vi "Wait on chirps generation - sweep.vi"(8 "error in (no error)":errorcluster) -> (0 "error out":errorcluster, 3 "Timed out waiting on Chirps generation":bool)   [LabVIEW 2017]
uses:
  Typedefs/Set Main VI cursor.ctl
  Global Variables/gl_UI Ctrl Refs.vi
  Global Variables/General Globals.vi
panel:
  out "Elapsed Time (s)":dbl
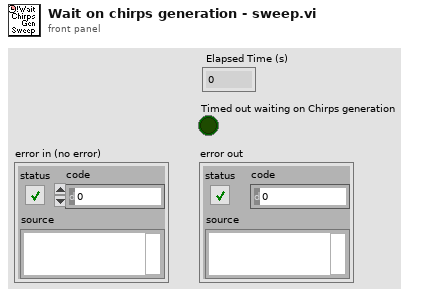
[diagram p1: front panel]
types:
  T1 = typedef "Set Main VI cursor.ctl" = enum16{"Release busy cursor", "Set busy cursor"}
  T2 = typedef "UI ctrl refs cluster.ctl" = cluster{"Top level VI path":path, "Top level VI ref":refnum<vi>, "User menu ref":refnum<k9>, "Sub Panel control":refnum<vi>, "Imaging Param Tab":refnum<vi>, "Occurrence-Start drivers":refnum<k4>, "Occurrence-Speed logging initialised":refnum<k4>, "Occurrence-XYZ stage initialised":refnum<k4>, "Exit button":refnum<vi>, "Status ind":refnum<vi>, "Set as origin":refnum<vi>, "Speed Logging":refnum<vi>, "Time Lapse":refnum<vi>, "Live Imaging":refnum<vi>, "AOL Z Stack":refnum<vi>, "Motor Z Stack":refnum<vi>, "Funct Acq button":refnum<vi>, "Hard Shutter":refnum<vi>, "Virtual Shutter":refnum<vi>, "Laser Power":refnum<vi>, "AOL Mode":refnum<vi>, "Frame Size":refnum<vi>, "Field of View":refnum<vi>, "Dwell Time":refnum<vi>, "Zoom":refnum<vi>, "AOL Z":refnum<vi>, "Objective":refnum<vi>, "Axis":refnum<vi>, "Paths & Names":refnum<vi>, "Experiment folder path (ind.)":refnum<vi>, "Last State (Ind.)":refnum<vi>, "Averages":refnum<vi>, "Angle (degrees)":refnum<vi>, "X centre":refnum<vi>, "Y centre":refnum<vi>, "Plane Mode":refnum<vi>, "# Planes":refnum<vi>, "Z Start":refnum<vi>, "Z Stop":refnum<vi>, "Z Step":refnum<vi>, "PMT 1":refnum<vi>, "PMT 2":refnum<vi>, "Stage XYZ Position":refnum<vi>, "Pockels@Z Start":refnum<vi>, "Pockels@Z Stop":refnum<vi>, "Obtain Z Start":refnum<vi>, "Obtain Z Stop":refnum<vi>, "Live stim.trig.period":refnum<vi>, "Live stim.trig.enable":refnum<vi>, "Movement Correction":refnum<vi>, "Load Reference Image":refnum<vi>, "XY Stage Move":refnum<vi>, "MovCor Cluster":refnum<vi>, "RefDAQParam":refnum<vi>, "Funct. Acq. Pockels Modulation":refnum<vi>, "Ref Laser Power":refnum<vi>, "Enable Video Recording":refnum<vi>, "Video Record-Live Imaging":refnum<vi>, "Video Record-Funct acq":refnum<vi>, "Reference Source":refnum<vi>, "AOL Z-stack Chirps Ready (ind)":refnum<vi>, "Target time between mov.cor. ref triggers (ms)":refnum<vi>, "Funct. Acq. Ref frame save":refnum<vi>, "Tracking button":refnum<vi>, "Show ref plots window":refnum<vi>, "Center freq ind (nm)":refnum<vi>, "Pickup mode (ind)":refnum<vi>, "Logging queue (ind)":refnum<vi>, "Back aperture power (ind.)":refnum<vi>, "Power after objective (ind.)":refnum<vi>, "Switch user":refnum<vi>, "Ls1 Conn. Status":refnum<vi>, "Ls1Tuning Status":refnum<vi>, "Ls1 Faults":refnum<vi>, "Ls1 Connection":refnum<vi>, "Ls1 Mode":refnum<vi>, "Ls1 POWER [mW]":refnum<vi>, "Ls1Shutter":refnum<vi>, "Ls1 Wavelength":refnum<vi>, "Ls1 Note":refnum<vi>, "Ls1 Confirm Wav":refnum<vi>, "Ls1 PreChrp Prism1":refnum<vi>, "Ls1 PreChrp Prism2":refnum<vi>, "Ls1 wav top Ind":refnum<vi>, "Ls1 power top Ind":refnum<vi>, "Ls1 Pump peak Hold":refnum<vi>, "Ls1 Status Ind":refnum<vi>, "Ls1 wav cancel":refnum<vi>, "Experiment Type":refnum<vi>, "Biology Information":refnum<vi>, "Camera recording status":refnum<vi>, "Start Sweep":refnum<vi>, "# Sw. Planes":refnum<vi>}
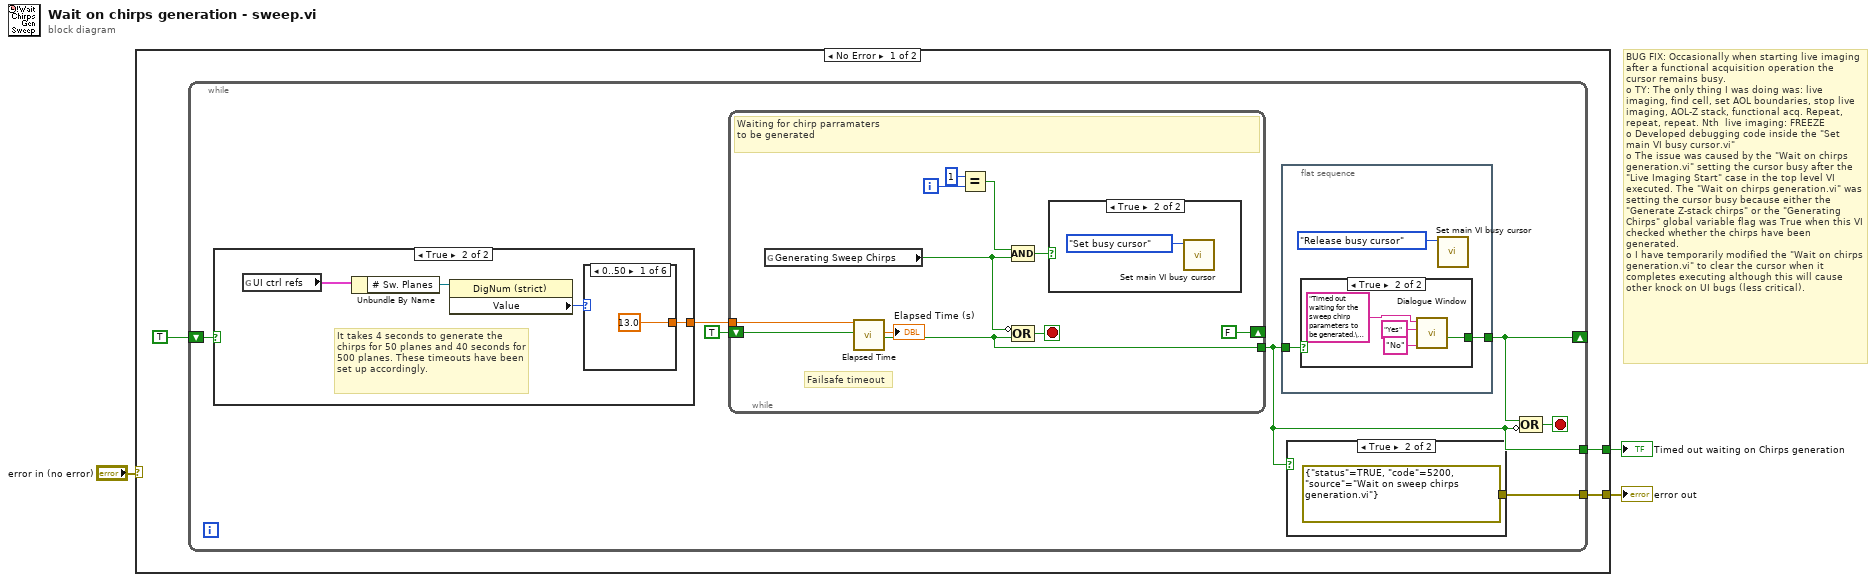
[diagram p0: block diagram]
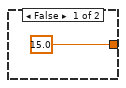
[diagram p3: hidden frame]
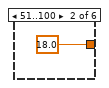
[diagram p4: hidden frame]
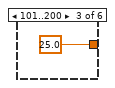
[diagram p5: hidden frame]
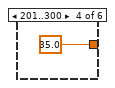
[diagram p6: hidden frame]
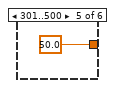
[diagram p7: hidden frame]
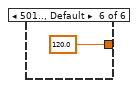
[diagram p8: hidden frame]
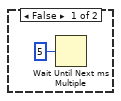
[diagram p10: hidden frame]
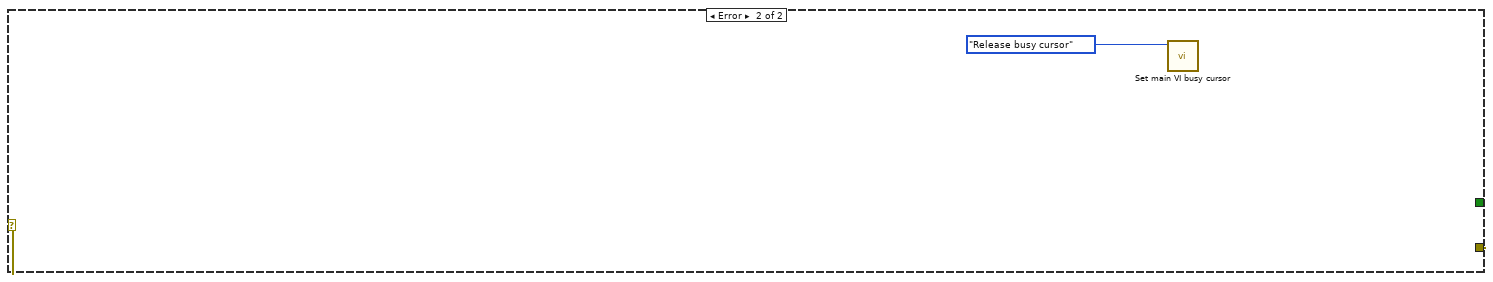
[diagram p11: hidden frame]
diagram:
  # "BUG FIX: Occasionally when starting live imaging after a functional acquisition operation the cursor remains busy.\no\tTY: The only thing I was doing was: live imaging, find cell, set AOL boundaries, stop live imaging, AOL-Z stack, functional acq. Repeat, repeat, repeat. Nth  live imaging: FREEZE\no\tDeveloped debugging code inside the \"Set main VI busy cursor.vi\"\no\tThe issue was caused by the \"Wait on chirps generation.vi\" setting the cursor busy after the \"Live Imaging Start\" case in the top level VI executed. The \"Wait on chirps generation.vi\" was setting the cursor busy because either the \"Generate Z-stack chirps\" or the \"Generating Chirps\" global variable flag was True when this VI checked whether the chirps have been generated.\no\tI have temporarily modified the \"Wait on chirps generation.vi\" to clear the cursor when it completes executing although this will cause other knock on UI bugs (less critical)."
  n1 = case shown="No Error" "error in (no error)" {
    selector: "error in (no error)" -> [_ w47]
    tunnel: [w4 w47] -> w2
    tunnel: [w6 _] -> w1
    frame No Error {
      n2 = while {
        tunnel: [w8] -> w6
        shift-right: [w7] -> _
        shift-left: TRUE -> [w10]
        tunnel: [w9] -> w4
        stop <- w11 stop-if-true
        n3 = case shown="True" w10 {
          tunnel: [15.0 ("Time Target (s)") w18] -> w12
          frame False {
          }
          frame True {
            # "It takes 4 seconds to generate the chirps for 50 planes and 40 seconds for 500 planes. These timeouts have been set up accordingly."
            n4 = global read "gl_UI Ctrl Refs.vi" "UI ctrl refs"() -> (w16:T2)
            n5 = Unbundle By Name(w16) -> ("# Sw. Planes"=w17:refnum<vi>)
            n6 = property class="DigNum (strict)"(reference=w17) -> ("Value"=w19:i32)  [unwired: 1 in, 2 out]
            n7 = case shown="0..50" w19 {
              tunnel: [13.0 ("Time Target (s)") 18.0 ("Time Target (s)") 25.0 ("Time Target (s)") 35.0 ("Time Target (s)") 50.0 ("Time Target (s)") 120.0 ("Time Target (s)")] -> w18
              frame 0..50 {
              }
              frame 51..100 {
              }
              frame 101..200 {
              }
              frame 201..300 {
              }
              frame 301..500 {
              }
              frame 501.., Default {
              }
            }
          }
        }
        n8 = while {
          shift-right: [FALSE] -> _
          shift-left: TRUE -> [w43]
          tunnel: [w40] -> w8
          tunnel: w12 -> [w34]
          i -> [w39]
          stop <- w41 stop-if-true
          # "Failsafe timeout"
          # "Waiting for chirp parramaters\nto be generated"
          n9 = global read "General Globals.vi" "Generating Sweep Chirps"() -> (w33:bool)
          n10 = call "Elapsed Time"("Time Target (s)"=w34, "Reset"=w43) -> ("Elapsed Time (s)"=→"Elapsed Time (s)":dbl, "Time has Elapsed"=w40:bool)  [unwired: 10 in, 6 out]
          n11 = Equal?(x=1, y=w39) -> (x = y?=w37:bool)
          n12 = Compound Arithmetic op=AND(w37, w33) -> (w36:bool)
          n13 = Compound Arithmetic op=OR(invert w33, w40) -> (w41:bool)
          n14 = case shown="True" w36 {
            frame False {
              n15 = Wait Until Next ms Multiple(millisecond multiple=u32 5) -> ()  [unwired: 1 out]
            }
            frame True {
              n16 = call "Set main VI busy cursor.vi"("Main VI's cursor"=Set_Main_VI_cursor."Set busy cursor") -> ()  [unwired: 10 in, 1 out]
            }
          }
        }
        n17 = flat-sequence {
          tunnel: w8 -> [w28]
          tunnel: [w27] -> w7
          frame #0 {
            n18 = case shown="True" w28 {
              tunnel: [_ w30] -> w27
              frame False {
              }
              frame True {
                n19 = call "Dialogue Window.vi"("Caption-Left button (Cancel)"="No", "Caption-Right button (OK)"="Yes", "Message string"="Timed out waiting for the sweep chirp parameters to be generated.\nWait a little longer?") -> ("Cancelled (Left button pressed)"=w30:bool)  [unwired: 6 in, 2 out]
              }
            }
            n20 = call "Set main VI busy cursor.vi"("Main VI's cursor"=Set_Main_VI_cursor."Release busy cursor") -> ()  [unwired: 10 in, 1 out]
          }
        }
        n21 = case shown="True" w8 {
          tunnel: [_ errorcluster {"status"=TRUE, "code"=5200, "source"="Wait on sweep chirps generation.vi"} ("error IO")] -> w9
          frame False {
          }
          frame True {
          }
        }
        n22 = Compound Arithmetic op=OR(w7, invert w8) -> (w11:bool)
      }
    }
    frame Error {
      n23 = call "Set main VI busy cursor.vi"("Main VI's cursor"=Set_Main_VI_cursor."Release busy cursor") -> ()  [unwired: 10 in, 1 out]
    }
  }
  "error out" <- w2
  "Timed out waiting on Chirps generation" <- w1
